vi "Get UDP Error Info.vi"(11 "error":T1) -> (2 "description":string, 3 "code":i32)   [LabVIEW 2017, in "UDP.lvlib" / "UDP Transceiver.lvclass"]
uses:
  UDP Transceiver.lvclass
  Errors.ctl
  Base Error Code.vi
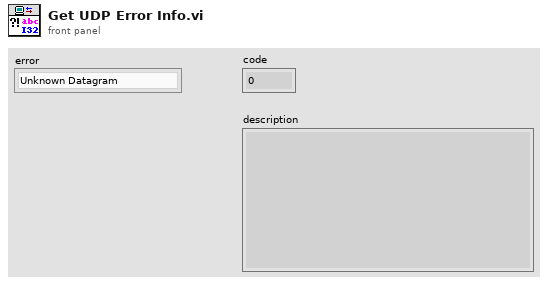
[diagram p1: front panel]
types:
  T1 = typedef "UDP.lvlib/UDP Transceiver.lvclass/Errors.ctl" = enum16{"Unknown Datagram", "Size Mismatch", "Invalid Setting"}
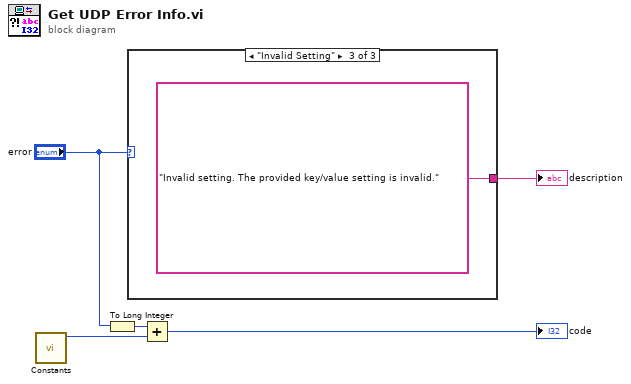
[diagram p0: block diagram]
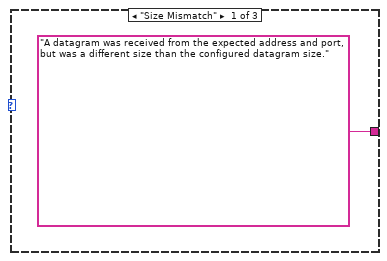
[diagram p2: hidden frame]
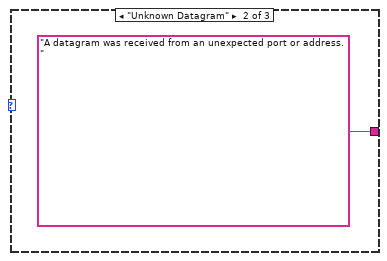
[diagram p3: hidden frame]
diagram:
  n1 = call-poly "Constants.vi"() -> ("base error code"=w5:i32)  [unwired: 11 in]
  n2 = To Long Integer(number="error") -> (32bit integer=w4:i32)
  n3 = case shown="\"Invalid Setting\"" "error" {
    tunnel: ["A datagram was received from the expected address and port, but was a different size than the configured datagram size." "A datagram was received from an unexpected port or address." "Invalid setting. The provided key/value setting is invalid."] -> w1
    frame "Size Mismatch" {
    }
    frame "Unknown Datagram" {
    }
    frame "Invalid Setting" {
    }
  }
  "description" <- w1
  n4 = Add(x=w4, y=w5) -> (x+y=→"code":i32)
